vi "UPdate Mask ROI List.vi"(8 "error in (no error)":errorcluster, 10 "MaskParam 2":refnum<vi>, 11 "Item Names":string[](array[string])) -> (0 "error out":errorcluster)   [LabVIEW 2019]
uses:
  Controls/MaskParam_Type.ctl
panel:
  out "Label.Text":string
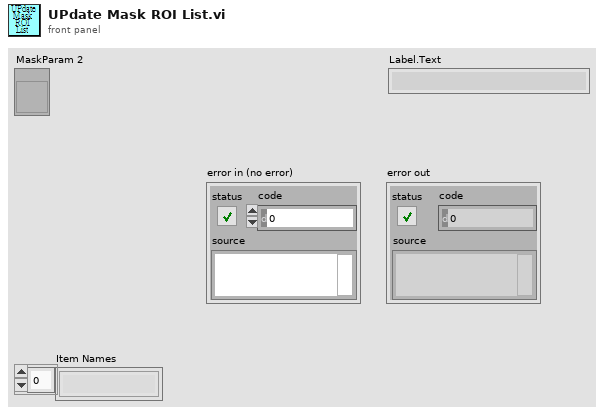
[diagram p1: front panel]
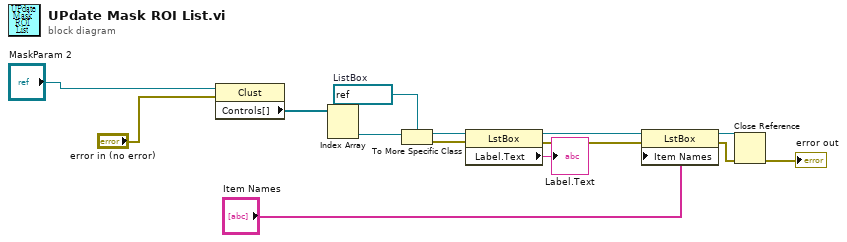
[diagram p0: block diagram]
diagram:
  w12 = refnum<vi> refnum  # ListBox
  n1 = property class="Clust"(reference="MaskParam 2", error in="error in (no error)") -> ("Controls[]"=w14:refnum<vi>[])  [unwired: 2 out]
  n2 = Index Array(array=w14) -> (element #2=w13:refnum<vi>)  [unwired: 2 in, 1 out]
  n3 = To More Specific Class(target class=w12, reference=w13) -> (specific class reference=w7:refnum<vi>, error out=w6:errorcluster)  [unwired: 1 in]
  n4 = property class="LstBox"(reference=w7, error in=w6) -> (reference out=w5:refnum<vi>, error out=w4:errorcluster, "Label.Text"=→"Label.Text":string)
  n5 = property class="LstBox"(reference=w5, error in=w4, "Item Names"="Item Names") -> (reference out=w9:refnum<vi>, error out=w10:errorcluster)
  n6 = Close Reference(reference=w9, error in (no error)=w10) -> (error out=→"error out":errorcluster)
